vi "Measuring Example (A).vi"() -> ()   [LabVIEW 2011]
uses:
  C:/Program Files/Metrohm Autolab/Autolab SDK 1.10/EcoChemie.Autolab.Sdk.dll
  EcoChemie.Autolab.Sdk.dll
panel:
  out "PotentialApplied":dbl
  in  "Embedded Exe File":path
  in  "Procedure":path=path "Standard Nova Procedures/Cyclic voltammetry.nox"
  in  "Load":bool
  in  "start measure":bool
  in  "Signal Y":string(combo)
  in  "Signal X":string(combo)
  in  "Abort":bool
  out "XY Graph":cluster{"Y":dbl[], "Y":dbl[]}[](graph)
  out "Value X":dbl
  out "IsMeasuring":bool
  out "Value Y":dbl
  in  "Save":bool
  in  "fileName":string
  in  "Stop":bool
  out "error out":errorcluster
  in  "Hardware Setup File":path
  out "IsConnected":bool
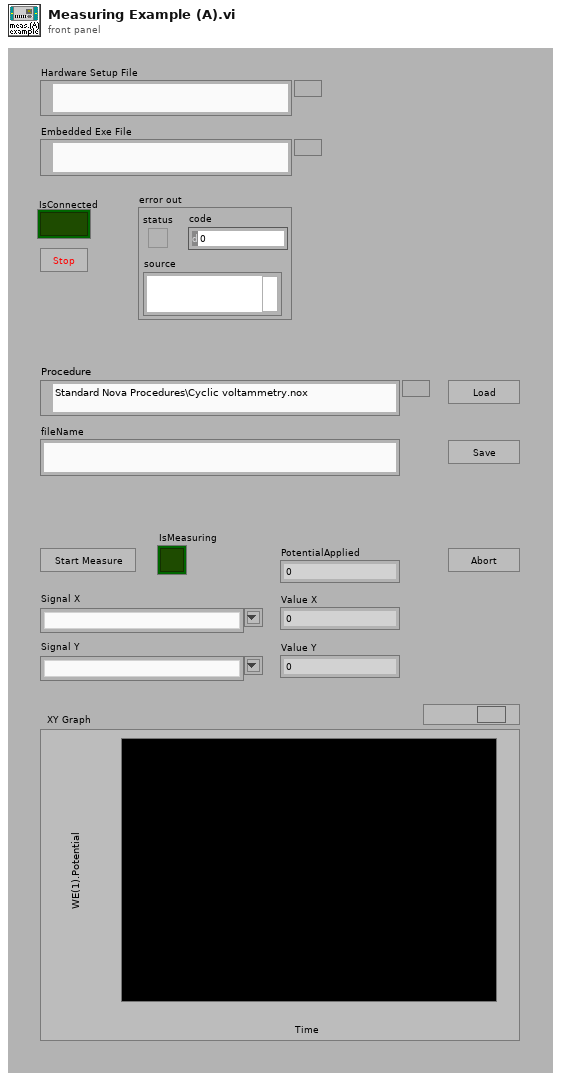
[diagram p1: front panel]
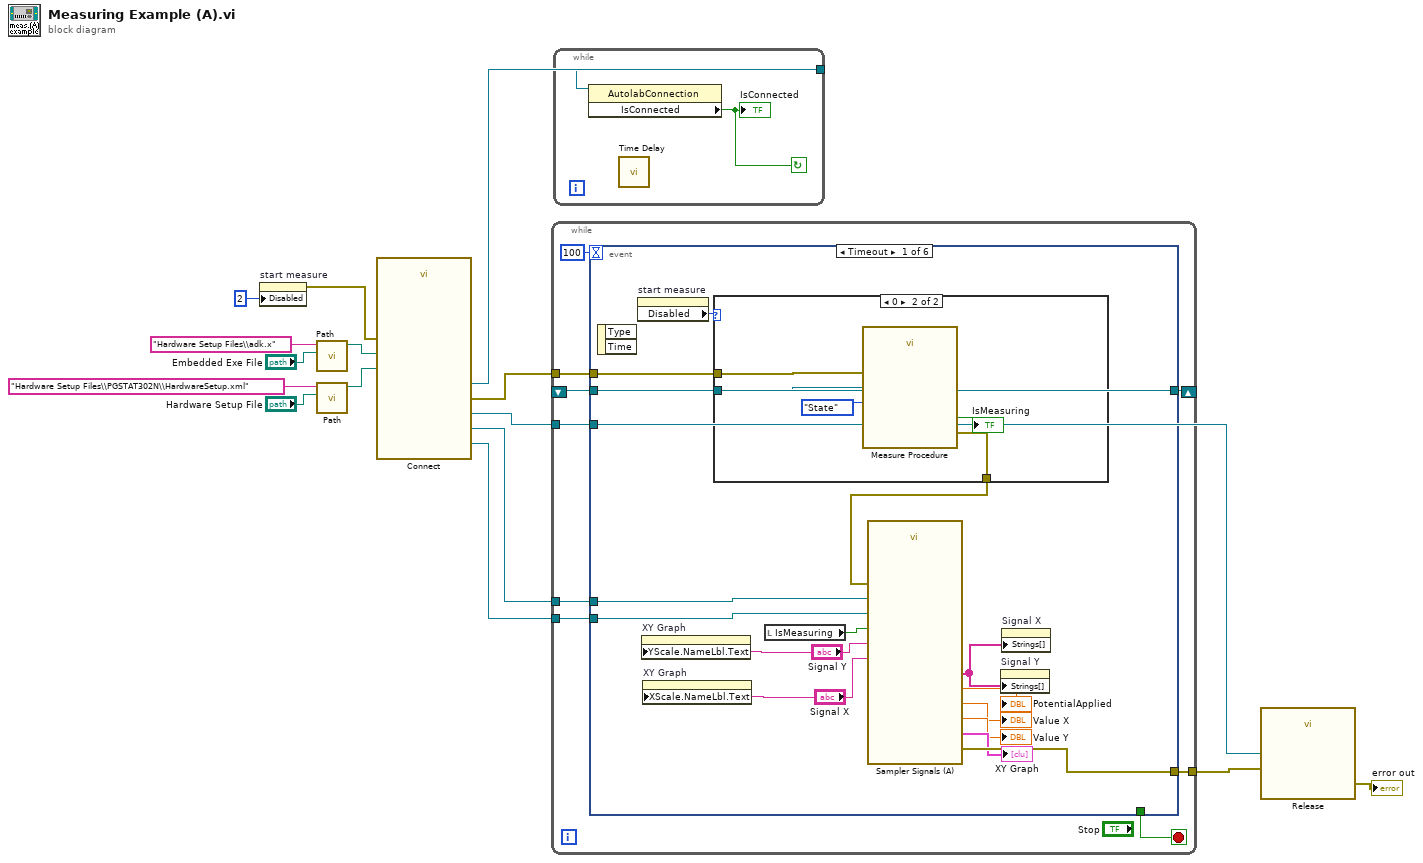
[diagram p0: block diagram]
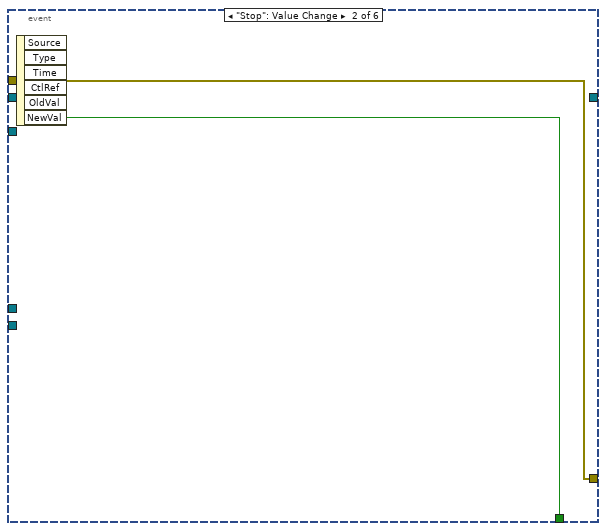
[diagram p3: hidden frame]
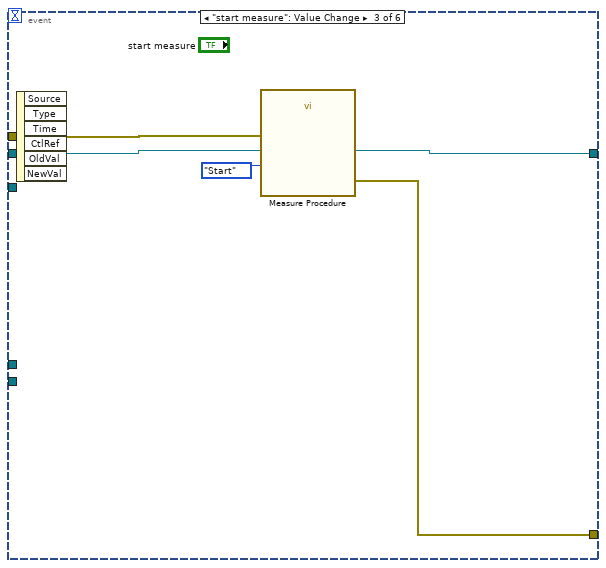
[diagram p4: hidden frame]
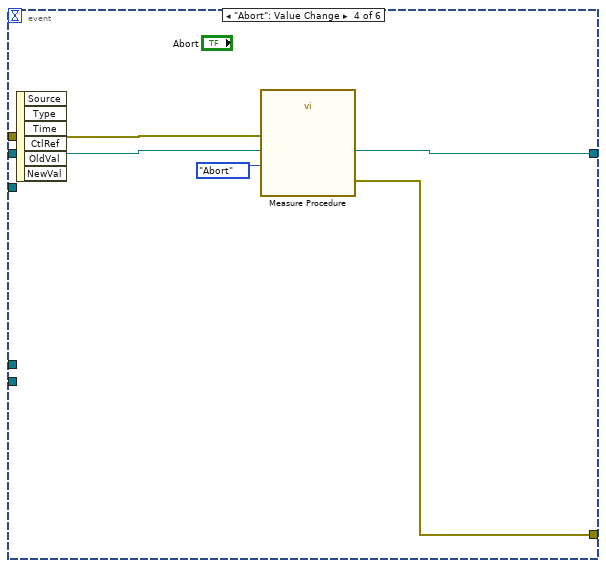
[diagram p5: hidden frame]
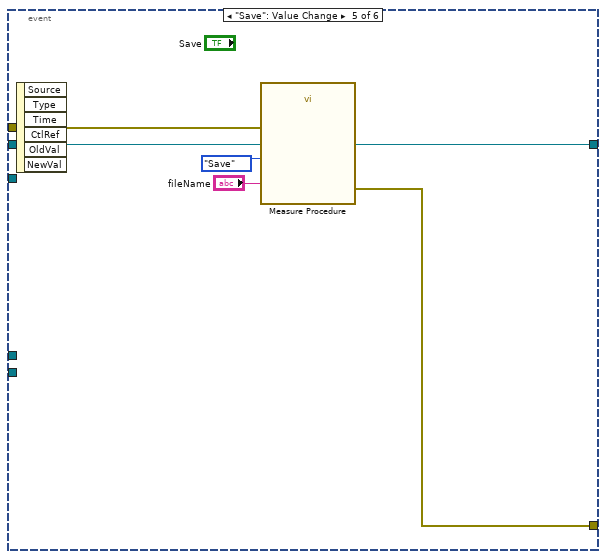
[diagram p6: hidden frame]
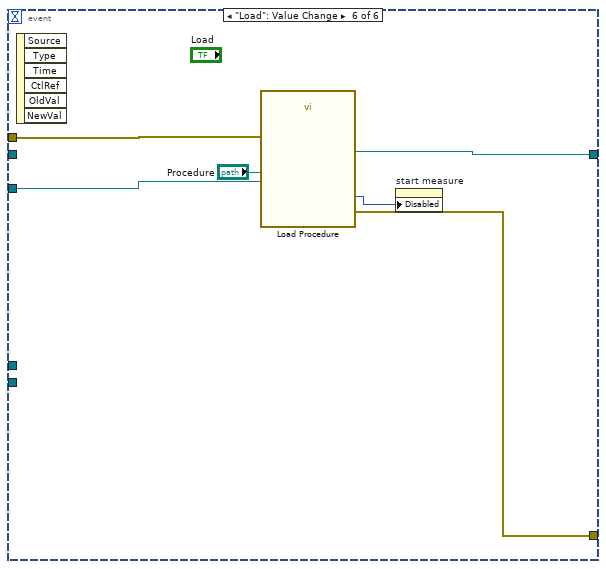
[diagram p7: hidden frame]
diagram:
  n1 = property on="start measure" class="Bool"("Disabled"=u8 2) -> (error out=w8:errorcluster)  [unwired: 2 in, 1 out]
  n2 = call "Path.vi"("File"="Embedded Exe File", "name or relative path"="Hardware Setup Files\\adk.x") -> ("appended path"=w2:path)  [unwired: 9 in]
  n3 = call "Path.vi"("File"="Hardware Setup File", "name or relative path"="Hardware Setup Files\\PGSTAT302N\\HardwareSetup.xml") -> ("appended path"=w1:path)  [unwired: 9 in]
  n4 = call "Connect.vi"("Embedded Exe File"=w2, "Hardware Setup File"=w1, "error in (no error)"=w8) -> ("Sampler"=w10:refnum<k24>, "AutolabConnection"=w14:refnum<k24>, "instrument"=w7:refnum<k24>, "Ei"=w11:refnum<k24>, "error out"=w12:errorcluster)  [unwired: 5 in, 3 out]
  n5 = while {
    shift-right: [w23] -> _
    shift-left: _ -> [w24]
    tunnel: w12 -> [w22]
    tunnel: w10 -> [w21]
    tunnel: w11 -> [w20]
    tunnel: [w19] -> w13
    tunnel: w7 -> [w17]
    stop <- w18 stop-if-true
    n6 = event shown="[0] Timeout" {
      selector: _ -> [_ _ _ _ _ _]
      dyn-events: _ -> [_ _ _ _ _ _]
      timeout: 100 -> [_ _ _ _ _ _]
      tunnel: w24 -> [w34 _ w49 w52 w59 _]
      tunnel: [w34 _ w49 w52 w59 w63] -> w23
      tunnel: w22 -> [w33 w46 w50 w54 w58 w62]
      tunnel: w21 -> [w37 _ _ _ _ _]
      tunnel: w20 -> [w36 _ _ _ _ _]
      tunnel: [w35 w46 w48 w53 w57 w61] -> w19
      tunnel: [_ w47 _ _ _ _] -> w18
      tunnel: w17 -> [_ _ _ _ _ w64]
      event Timeout {
        n7 = event-data() -> ()  [unwired: 1 in, 2 out]
        n8 = property on="start measure" class="Bool"() -> ("Disabled"=w39:u8)  [unwired: 2 in, 2 out]
        n9 = property on="XY Graph" class="XYGraph (strict)"("YScale.NameLbl.Text"="Signal Y") -> ()  [unwired: 2 in, 2 out]
        n10 = property on="XY Graph" class="XYGraph (strict)"("XScale.NameLbl.Text"="Signal X") -> ()  [unwired: 2 in, 2 out]
        n11 = case shown="0" w39 {
          tunnel: w34 -> [_ w41]
          tunnel: w33 -> [w40 w42]
          tunnel: [w40 w43] -> w38
          frame 2, Default {
          }
          frame 0 {
            n12 = call "Measure Procedure.vi"("error in"=w42, "Request for procedure"=enum16{"State", "Save", "Abort", "Start"}."State", "LoadProcedure"=w41) -> ("error out"=w43:errorcluster, "IsMeasuring"=→"IsMeasuring":bool)  [unwired: 7 in]
          }
        }
        n13 = local read "IsMeasuring"() -> (w32:bool)
        n14 = call "Sampler Signals (A).vi"("IsMeasuring"=w32, "EI"=w36, "Sampler"=w37, "Signal X"="Signal X", "Signal Y"="Signal Y", "error in"=w38) -> ("PotentialApplied"=→"PotentialApplied":dbl, "X"=→"Value X":dbl, "Y"=→"Value Y":dbl, "XY Graph"=→"XY Graph":cluster{"Y":dbl[], "Y":dbl[]}[], "GetSignals"=w25:string[], "error out"=w35:errorcluster)  [unwired: 4 in]
        n15 = property on="Signal Y" class="CmbBox"("Strings[]"=w25) -> ()  [unwired: 2 in, 2 out]
        n16 = property on="Signal X" class="CmbBox"("Strings[]"=w25) -> ()  [unwired: 2 in, 2 out]
      }
      event "Stop": Value Change {
        n17 = event-data() -> ("NewVal"=w47:bool)  [unwired: 1 in, 5 out]
      }
      event "start measure": Value Change {
        n18 = event-data() -> ()  [unwired: 1 in, 6 out]
        n19 = call "Measure Procedure.vi"("error in"=w50, "Request for procedure"=enum16{"State", "Save", "Abort", "Start"}."Start", "LoadProcedure"=w49) -> ("error out"=w48:errorcluster)  [unwired: 7 in, 1 out]
      }
      event "Abort": Value Change {
        n20 = event-data() -> ()  [unwired: 1 in, 6 out]
        n21 = call "Measure Procedure.vi"("error in"=w54, "Request for procedure"=enum16{"State", "Save", "Abort", "Start"}."Abort", "LoadProcedure"=w52) -> ("error out"=w53:errorcluster)  [unwired: 7 in, 1 out]
      }
      event "Save": Value Change {
        n22 = event-data() -> ()  [unwired: 1 in, 6 out]
        n23 = call "Measure Procedure.vi"("error in"=w58, "fileName"="fileName", "Request for procedure"=enum16{"State", "Save", "Abort", "Start"}."Save", "LoadProcedure"=w59) -> ("error out"=w57:errorcluster)  [unwired: 6 in, 1 out]
      }
      event "Load": Value Change {
        n24 = event-data() -> ()  [unwired: 1 in, 6 out]
        n25 = call "Load Procedure.vi"("error in (no error)"=w62, "Procedure"="Procedure", "Instrument"=w64) -> ("error out"=w61:errorcluster, "Numeric"=w66:i32, "LoadProcedure"=w63:refnum<k24>)  [unwired: 5 in, 1 out]
        n26 = property on="start measure" class="Bool"("Disabled"=w66) -> ()  [unwired: 2 in, 2 out]
      }
    }
  }
  n27 = while {
    tunnel: w14 -> [w68]
    stop <- w67 continue-if-true
    n28 = property class="AutolabConnection"(reference=w68) -> ("IsConnected"=w67:bool)  [unwired: 1 in, 2 out]
    "IsConnected" <- w67
    n29 = call "Time Delay"() -> ()  [unwired: 11 in, 1 out]
  }
  n30 = call "Release.vi"("error in (no error)"=w13, "Instrument"=w7) -> ("error out"=→"error out":errorcluster)  [unwired: 9 in]
